vi "Script Test.vi"(0 "Image In":T1, 7 "error in":errorcluster) -> (20 "Image Out":T1, 27 "error out":errorcluster)   [LabVIEW 2015]
uses:
  <vilib>/vision/Image Controls.llb/IMAQ Image.ctl
  <vilib>/vision/NI_Vision_Development_Module.lvlib
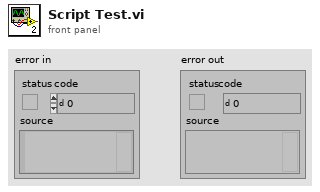
[diagram p1: front panel]
types:
  T1 = typedef "IMAQ Image.ctl" = refnum<image>
  T2 = cluster{"Pos. X":i32, "Pos. Y":i32, "Radius":i32, "Core Area":i32}[]
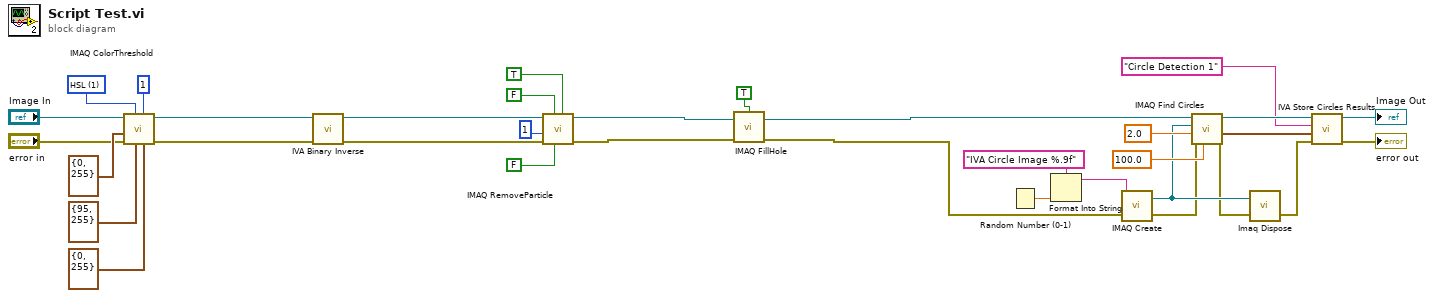
[diagram p0: block diagram]
diagram:
  w32 = u16 1 items=["RGB", "HSL", "HSV", "HSI"] ("Color Mode")
  n1 = call "IMAQ ColorThreshold"("Blue or Luma or Val or Inten Range"=cluster{"Lower value":i32, "Upper value":i32} {"Lower value"=0, "Upper value"=255}, "Replace Value"=1, "Green or Sat Range"=cluster{"Lower value":i32, "Upper value":i32} {"Lower value"=95, "Upper value"=255}, "Color Mode"=w32, "error in (no error)"="error in", "Red or Hue Range"=cluster{"Lower value":i32, "Upper value":i32} {"Lower value"=0, "Upper value"=255}, "Image Src"="Image In") -> ("error out"=w26:errorcluster, "Image Dst Out"=w25:T1)  [unwired: 1 in, 2 out]
  n2 = call <vilib>:"IVA Binary Inverse.vi"("error in (no error)"=w26, "Image In"=w25) -> ("error out"=w24:errorcluster, "Image Out"=w19:T1)  [unwired: 8 out]
  n3 = call "IMAQ RemoveParticle"("Connectivity 4/8 (8)"=TRUE, "Low Pass/High Pass (Low)"=FALSE, "Square/Hexa (Square)"=FALSE, "error in (no error)"=w24, "Number of Erosion"=1, "Image Src"=w19) -> ("error out"=w18:errorcluster, "Image Dst Out"=w16:T1)  [unwired: 1 in, 3 out]
  n4 = call "IMAQ FillHole"("error in (no error)"=w18, "Image Src"=w16, "Connectivity 4/8 (8)"=TRUE) -> ("error out"=w15:errorcluster, "Image Dst Out"=w7:T1)  [unwired: 1 in, 2 out]
  n5 = Random Number (0-1)() -> (number: 0 to 1=w1:dbl)
  n6 = Format Into String(format string="IVA Circle Image %.9f" ("Image Name"), w1) -> (resulting string=w3:string)  [unwired: 2 in, 1 out]
  n7 = call "IMAQ Create"("Image Name"=w3, "error in (no error)"=w15) -> ("New Image"=w12:T1, "error out"=w11:errorcluster)  [unwired: 2 in, 1 out]
  n8 = call "IMAQ Find Circles"("Max Radius"=sgl 100.0, "error in (no error)"=w11, "Min Radius"=sgl 2.0, "Image Dst"=w12, "Image Src"=w7) -> ("error out"=w10:errorcluster, "Circles Data"=w4:T2)  [unwired: 5 out]
  n9 = call "Imaq Dispose"("Image"=w12, "error in (no error)"=w10) -> ("error out"=w9:errorcluster)  [unwired: 1 in, 3 out]
  n10 = call <vilib>:"IVA Store Circles Results.vi"("error in (no error)"=w9, "Circles Data"=w4, "Step Name"="Circle Detection 1", "Image in"=w7) -> ("error out"=→"error out":errorcluster, "Image dup"=→"Image Out":T1)  [unwired: 6 out]
